vi "Read Periodic Delay Parameters.vi"(11 "User Interface in":refnum<class "User Interface.lvclass">) -> (2 "Periodic Delay Parameters":refnum<vi>, 3 "User Interface out":refnum<class "User Interface.lvclass">)   [LabVIEW 2016, in "_User Interface.lvlib" / "User Interface.lvclass"]
uses:
  User Interface.lvclass
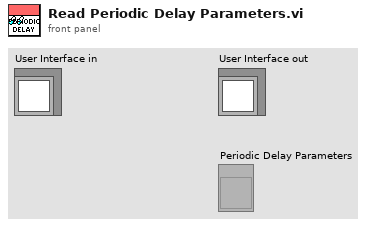
[diagram p1: front panel]
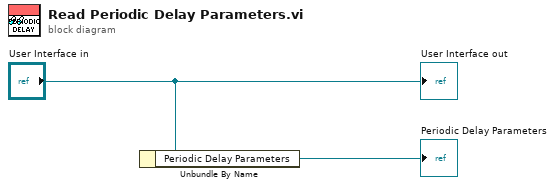
[diagram p0: block diagram]
diagram:
  n1 = Unbundle By Name("User Interface in") -> ("Periodic Delay Parameters"=→"Periodic Delay Parameters":refnum<vi>)
  "User Interface out" <- "User Interface in"
